vi "Transistor curve.vi"() -> ()   [LabVIEW 2014]
uses:
  Environmental Chamber LabVIEW and Instruments/Drivers and Software/LabVIEW 8.2 Drivers/keithley_24xx/Keithley 24XX/Public/Data/Read (Single Point).vi
  <vilib>/Utility/file.llb/Write To Spreadsheet File (string).vi
  Environmental Chamber LabVIEW and Instruments/Drivers and Software/keithley_24xx/Keithley 24XX/Keithley 24XX.lvlib
  Environmental Chamber LabVIEW and Instruments/Drivers and Software/keithley_6430/Keithley 6430/Keithley 6430.lvlib
panel:
  in  "# of curves":i16
  in  "Delay (s)":dbl
  in  "Bias (V)":dbl
  in  "voltage settings":T1={"Vi (V)"=0.0, "Vf (V)"=0.3, "# of points"=30.0}
  out "File path":path
  in  "STOP":bool
  out "V":dbl
  out "2420 IV curve":cluster{"X":dbl[], "Y":dbl[]}[](graph)
  out "I":sgl
  out "R":sgl
  in  "File notes":string
  # "6430 = bias\n2420 = source-drain"
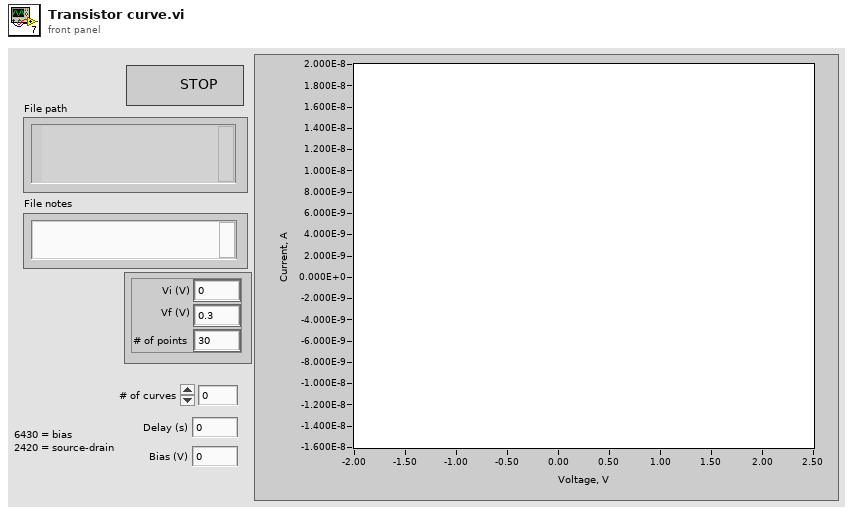
[diagram p1: front panel]
types:
  T1 = cluster{"Vi (V)":dbl, "Vf (V)":dbl, "# of points":dbl}
  T2 = enum16{"open", "replace", "create", "open or create", "replace or create", "replace or create with confirmation"}
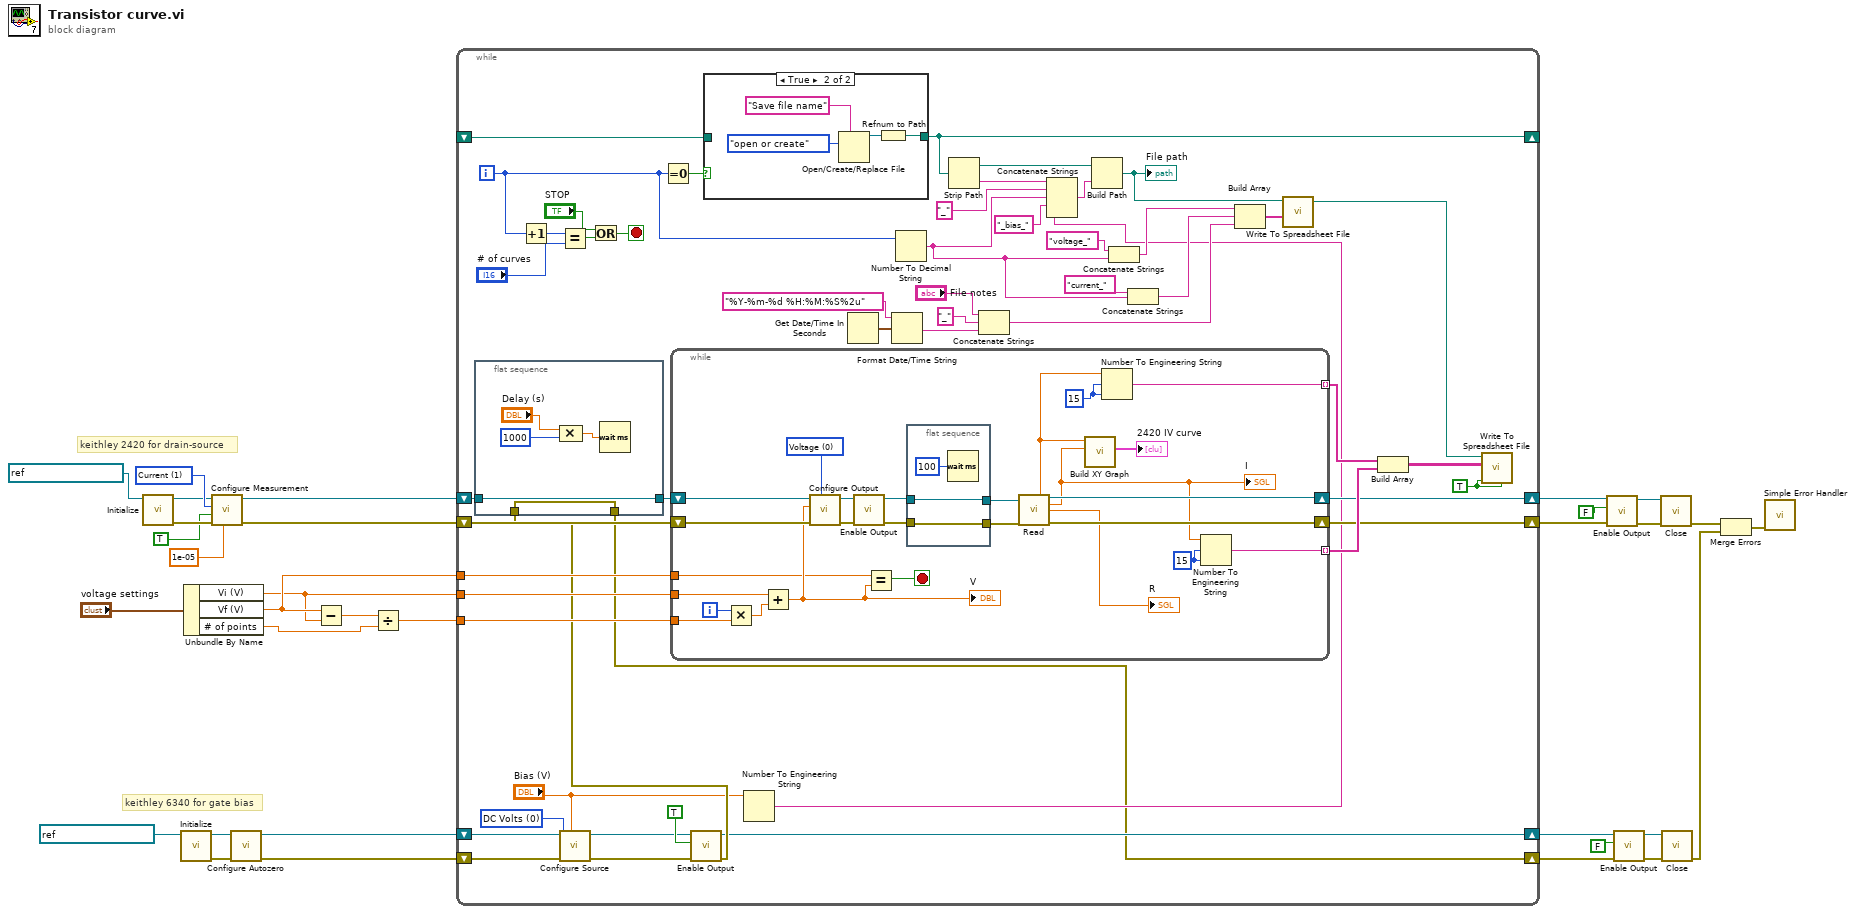
[diagram p0: block diagram]
diagram:
  w24 = u16 1 items=["Volts", "Current", "Resistance"] ("Function (0: Volts)")
  # "keithley 6340 for gate bias"
  # "keithley 2420 for drain-source"
  n1 = call "Initialize.vi"("VISA resource name"=refnum<visa-resource-name> "GPIB1::24::INSTR") -> ("error out"=w20:errorcluster, "VISA resource name out"=w21:refnum<visa-resource-name>)  [unwired: 9 in]
  n2 = call "Initialize.vi"("VISA resource name"=refnum<visa-resource-name> "GPIB0::29::INSTR") -> ("error out"=w11:errorcluster, "VISA resource name out"=w12:refnum<visa-resource-name>)  [unwired: 4 in, 5 out]
  n3 = Unbundle By Name("voltage settings") -> ("Vi (V)"=w14:dbl, "Vf (V)"=w15:dbl, "# of points"=w16:dbl)
  n4 = call "Configure Measurement.vi"("Manual Range (1.0)"=1e-05, "error in (no error)"=w20, "Enable Auto Range (T:Enable)"=TRUE, "Function (0: Volts)"=w24, "VISA resource name"=w21) -> ("error out"=w23:errorcluster, "VISA resource name out"=w22:refnum<visa-resource-name>)  [unwired: 5 in]
  n5 = call "Configure Autozero.vi"("error in (no error)"=w11, "VISA resource name"=w12) -> ("error out"=w1:errorcluster, "VISA resource name out"=w2:refnum<visa-resource-name>)  [unwired: 8 in]
  n6 = Subtract(x=w15, y=w14) -> (x-y=w32:dbl)
  n7 = Divide(x=w32, y=w16) -> (x/y=w31:dbl)
  n8 = while {
    tunnel: w15 -> [w83]
    tunnel: w14 -> [w82]
    tunnel: w31 -> [w81]
    shift-right: [w73] -> w26
    shift-left: w23 -> [w72]
    shift-right: [w74] -> w27
    shift-left: w22 -> [w53]
    shift-right: [w62] -> _
    shift-left: _ -> [w63]
    shift-right: [w33] -> w6
    shift-left: w1 -> [w42]
    shift-right: [w34] -> w7
    shift-left: w2 -> [w43]
    i -> [w65]
    stop <- w69 stop-if-true
    w45 = u16 0 items=["DC Volts", "DC Current"] ("Source Function (0: DC Volts)")
    w80 = TRUE ("transpose? (no:F)")
    n9 = flat-sequence {
      tunnel: [w88] -> w52
      tunnel: w53 -> [w88]
      tunnel: w39 -> [w85]
      tunnel: [w85] -> w33
      frame #0 {
        n10 = Compound Arithmetic op=MULTIPLY("Delay (s)", u32 1000 ("value")) -> (w87:dbl)
        n11 = Wait (ms)(milliseconds to wait=w87) -> ()  [unwired: 1 out]
      }
    }
    n12 = Increment(x=w65) -> (x+1=w67:i32)
    n13 = Equal?(x=w67, y="# of curves") -> (x = y?=w66:bool)
    n14 = call "Configure Source.vi"("V-Source Level [V]"="Bias (V)", "error in (no error)"=w42, "Source Function (0: DC Volts)"=w45, "VISA resource name"=w43) -> ("error out"=w35:errorcluster, "VISA resource name out"=w36:refnum<visa-resource-name>)  [unwired: 6 in]
    n15 = Or(x="STOP", y=w66) -> (x .or. y?=w69:bool)
    n16 = Equal To 0?(x=w65) -> (x = 0?=w64:bool)
    n17 = while {
      tunnel: [w112] -> w76 mode=indexing
      shift-right: [w118] -> w73
      shift-left: w72 -> [w117]
      shift-right: [w119] -> w74
      shift-left: w52 -> [w116]
      tunnel: w81 -> [w94]
      tunnel: w82 -> [w107]
      tunnel: [w106] -> w77 mode=indexing
      tunnel: w83 -> [w96]
      i -> [w95]
      stop <- w98 stop-if-true
      w102 = i16 15 ("precision (6)")
      w103 = i16 15 ("precision (6)")
      w113 = u16 0 items=["Voltage", "Current"] ("Source Mode  (0: Voltage)")
      n18 = Multiply(x=w95, y=w94) -> (x*y=w105:dbl)
      n19 = Add(x=w107, y=w105) -> (x+y=w97:dbl)
      "V" <- w97
      n20 = call "Configure Output.vi"("Source Mode  (0: Voltage)"=w113, "error in (no error)"=w117, "Output Level (0)"=w97, "VISA resource name"=w116) -> ("error out"=w115:errorcluster, "VISA resource name out"=w114:refnum<visa-resource-name>)  [unwired: 6 in]
      n21 = call "Enable Output.vi"("error in (no error)"=w115, "VISA resource name"=w114) -> ("error out"=w108:errorcluster, "VISA resource name out"=w111:refnum<visa-resource-name>)  [unwired: 8 in]
      n22 = Equal?(x=w96, y=w97) -> (x = y?=w98:bool)
      n23 = flat-sequence {
        tunnel: [w122] -> w110
        tunnel: w111 -> [w122]
        tunnel: w108 -> [w121]
        tunnel: [w121] -> w109
        frame #0 {
          n24 = Wait (ms)(milliseconds to wait=u32 100) -> ()  [unwired: 1 out]
        }
      }
      n25 = call-poly "Read.vi"("VISA resource name"=w110, "error in (no error)"=w109) -> ("Voltage"=w100:sgl, "VISA resource name out"=w119:refnum<visa-resource-name>, "Current"=w101:sgl, "Resistance"=→"R":sgl, "error out"=w118:errorcluster)  [unwired: 7 in, 2 out]
      "I" <- w101
      n26 = call "Build XY Graph"("Y Input"=w101, "X Input"=w100) -> ("XY Graph"=→"2420 IV curve":cluster{"X":dbl[], "Y":dbl[]}[])  [unwired: 8 in, 1 out]
      n27 = Number To Engineering String(2:w102, 3:w102, 4:w100) -> (0:w106:string)  [unwired: 1 in]
      n28 = Number To Engineering String(2:w103, 3:w103, 4:w101) -> (0:w112:string)  [unwired: 1 in]
    }
    n29 = call "Enable Output.vi"("error in (no error)"=w35, "Enable Output (F:Off)"=TRUE ("Output (F:Off)"), "VISA resource name"=w36) -> ("error out"=w39:errorcluster, "VISA resource name out"=w34:refnum<visa-resource-name>)  [unwired: 7 out]
    n30 = case shown="True" w64 {
      tunnel: [w89 w90] -> w62
      tunnel: w63 -> [w89 _]
      frame False {
      }
      frame True {
        n31 = Open/Create/Replace File(prompt="Save file name", operation (0:open)=T2."open or create") -> (refnum out=w91:refnum<file>)  [unwired: 4 in, 2 out]
        n32 = Refnum to Path(1:w91) -> (0:w90:path)
      }
    }
    n33 = Number To Engineering String(4:"Bias (V)") -> (0:w40:string)  [unwired: 3 in]
    n34 = Get Date/Time In Seconds() -> (seconds since 1Jan1904=w58:timestamp)
    n35 = Format Date/Time String(time format string (%c)="%Y-%m-%d %H:%M:%S%2u", seconds (now)=w58) -> (date/time string=w54:string)  [unwired: 1 in]
    n36 = Number To Decimal String(number=w65) -> (decimal integer string=w48:string)  [unwired: 1 in]
    n37 = Strip Path(path=w62) -> (stripped path=w61:path, name=w60:string)
    n38 = Concatenate Strings("File notes", "_" ("string"), w54) -> (w55:string)
    n39 = Concatenate Strings(w60, "_" ("string"), w48, "_bias_", w40) -> (w51:string)
    n40 = Build Path(base path=w61, name or relative path=w51) -> (appended path=w71:path)
    "File path" <- w71
    n41 = Concatenate Strings("voltage_", w48) -> (w46:string)
    n42 = Concatenate Strings("current_", w48) -> (w49:string)
    n43 = Build Array(w46, w49, w55) -> (w79:string[])
    n44 = call-poly <vilib>:"Write To Spreadsheet File.vi"("1D data"=w79, "file path (dialog if empty)"=w71) -> ("new file path (Not A Path if cancelled)"=w78:path)  [unwired: 6 in]
    n45 = Build Array(w77, w76) -> (w75:string[][])
    n46 = call-poly <vilib>:"Write To Spreadsheet File.vi"("transpose? (no:F)"=w80, "append to file? (new file:F)"=w80, "2D data"=w75, "file path (dialog if empty)"=w78) -> ()  [unwired: 4 in, 1 out]
  }
  n47 = call "Enable Output.vi"("error in (no error)"=w26, "Enable Output (T: Enable)"=FALSE, "VISA resource name"=w27) -> ("error out"=w28:errorcluster, "VISA resource name out"=w30:refnum<visa-resource-name>)  [unwired: 7 in]
  n48 = call "Enable Output.vi"("error in (no error)"=w6, "Enable Output (F:Off)"=FALSE ("Output (F:Off)"), "VISA resource name"=w7) -> ("error out"=w8:errorcluster, "VISA resource name out"=w9:refnum<visa-resource-name>)  [unwired: 7 out]
  n49 = call "Close.vi"("error in (no error)"=w28, "VISA resource name"=w30) -> ("error out"=w5:errorcluster)  [unwired: 9 in]
  n50 = call "Close.vi"("error in (no error)"=w8, "VISA resource name"=w9) -> ("error out"=w4:errorcluster)  [unwired: 9 out]
  n51 = Merge Errors(w5, w4) -> (w3:errorcluster)
  n52 = call <vilib>:"Simple Error Handler.vi"("error in (no error)"=w3) -> ()  [unwired: 4 in, 5 out]
